vi "dds writer config to reader.vi"(11 "writer configuration":T1) -> (3 "reader configuration":T2)   [LabVIEW 2014, in "DDS configuration.lvclass"]
uses:
  DDS configuration.lvclass
  <vilib>/RTI DDS Toolkit for LabVIEW/Types/RTI DDS Advanced Reader Configuration.ctl
  <vilib>/RTI DDS Toolkit for LabVIEW/Types/RTI DDS Advanced Writer Configuration.ctl
  <vilib>/RTI DDS Toolkit for LabVIEW/Library/LVDDS_library.lvlib
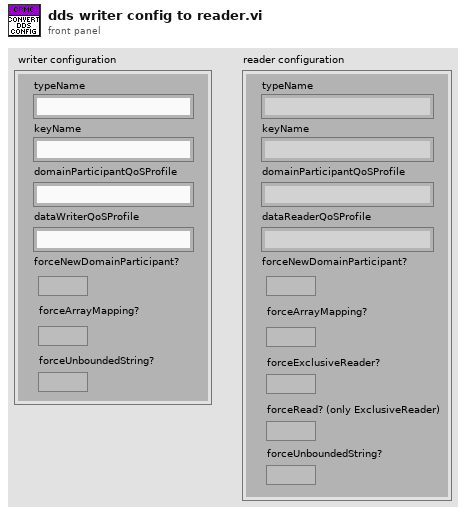
[diagram p1: front panel]
types:
  T1 = typedef "LVDDS_library.lvlib/RTI DDS Advanced Writer Configuration.ctl" = cluster{"typeName":string, "keyName":string, "domainParticipantQoSProfile":string, "dataWriterQoSProfile":string, "forceNewDomainParticipant?":bool, "forceArrayMapping?":bool, "forceUnboundedString?":bool}
  T2 = typedef "LVDDS_library.lvlib/RTI DDS Advanced Reader Configuration.ctl" = cluster{"typeName":string, "keyName":string, "domainParticipantQoSProfile":string, "dataReaderQoSProfile":string, "forceNewDomainParticipant?":bool, "forceArrayMapping?":bool, "forceExclusiveReader?":bool, "forceRead? (only ExclusiveReader)":bool, "forceUnboundedString?":bool}
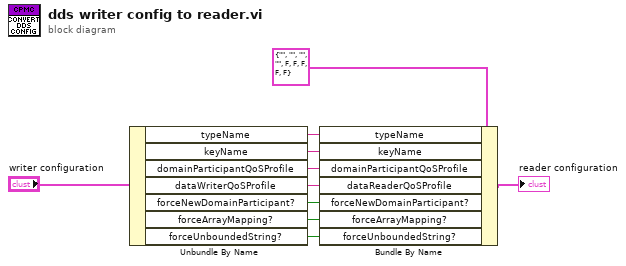
[diagram p0: block diagram]
diagram:
  n1 = Unbundle By Name("writer configuration") -> ("typeName"=w10:string, "keyName"=w9:string, "domainParticipantQoSProfile"=w8:string, "dataWriterQoSProfile"=w7:string, "forceNewDomainParticipant?"=w6:bool, "forceArrayMapping?"=w5:bool, "forceUnboundedString?"=w4:bool)
  n2 = Bundle By Name(cluster=T2 {"typeName"="", "keyName"="", "domainParticipantQoSProfile"="", "dataReaderQoSProfile"="", "forceNewDomainParticipant?"=FALSE, "forceArrayMapping?"=FALSE, "forceExclusiveReader?"=FALSE, "forceRead? (only ExclusiveReader)"=FALSE, "forceUnboundedString?"=FALSE} ("reader configuration"), "typeName"=w10, "keyName"=w9, "domainParticipantQoSProfile"=w8, "dataReaderQoSProfile"=w7, "forceNewDomainParticipant?"=w6, "forceArrayMapping?"=w5, "forceUnboundedString?"=w4) -> (→"reader configuration":T2)
